vi "GetStatus.vi"(8 "error in":errorcluster, 10 "Status":string, 11 "VISA resource name":refnum<visa-resource-name>) -> (0 "error out":errorcluster, 3 "VISA resource name out":refnum<visa-resource-name>)   [LabVIEW 2017, in "TCxxxx.lvlib"]
uses:
  TCxxxx.lvlib
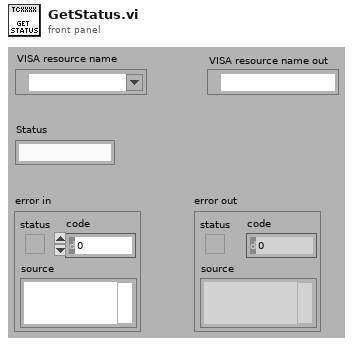
[diagram p1: front panel]
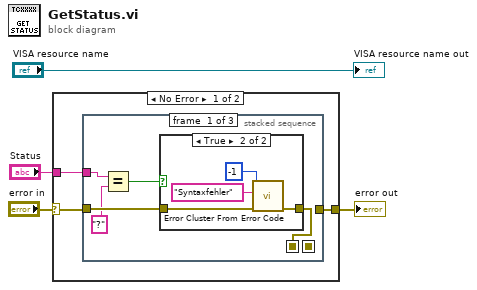
[diagram p0: block diagram]
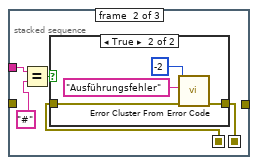
[diagram p3: hidden frame]
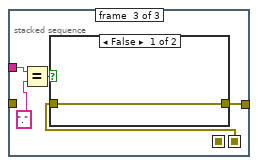
[diagram p5: hidden frame]
diagram:
  n1 = case shown="No Error" "error in" {
    selector: "error in" -> [w6 w35]
    tunnel: [w7 w35] -> w3
    tunnel: "Status" -> [w5 _]
    frame No Error {
      n2 = stacked-sequence {
        seq-local: [w8 _ _] -> [_ w19 _]
        seq-local: [_ w18 _] -> [_ _ w29]
        tunnel: w6 -> [w12 _ _]
        tunnel: [_ _ w28] -> w7
        tunnel: w5 -> [w10 w21 w31]
        frame #0 {
          n3 = Equal?(x=w10, y="?") -> (x = y?=w11:bool)
          n4 = case shown="True" w11 {
            tunnel: w12 -> [w13 w17]
            tunnel: [w13 w14] -> w8
            frame False {
            }
            frame True {
              n5 = call <vilib>:"Error Cluster From Error Code.vi"("error in (no error)"=w17, "error message (\"\")"="Syntaxfehler" ("error message (\"\")"), "error code (0)"=-1) -> ("error out"=w14:errorcluster)  [unwired: 6 in]
            }
          }
        }
        frame #1 {
          n6 = Equal?(x=w21, y="#") -> (x = y?=w22:bool)
          n7 = case shown="True" w22 {
            tunnel: w19 -> [w23 w27]
            tunnel: [w23 w24] -> w18
            frame False {
            }
            frame True {
              n8 = call <vilib>:"Error Cluster From Error Code.vi"("error in (no error)"=w27, "error message (\"\")"="Ausführungsfehler" ("error message (\"\")"), "error code (0)"=-2) -> ("error out"=w24:errorcluster)  [unwired: 6 in]
            }
          }
        }
        frame #2 {
          n9 = Equal?(x=w31, y=".") -> (x = y?=w32:bool)
          n10 = case shown="False" w32 {
            tunnel: w29 -> [w33 w34]
            tunnel: [w33 w34] -> w28
            frame False {
            }
            frame True {
            }
          }
        }
      }
    }
    frame Error {
    }
  }
  "error out" <- w3
  "VISA resource name out" <- "VISA resource name"
